vi "Helmholtz2D_FEM_Solve U.vi"(8 "error in (no error)":errorcluster, 11 "Helmholtz2D FEM Data In":T1) -> (0 "error out":errorcluster, 3 "Helmholtz2D FEM Data Out":T1)   [LabVIEW 2017, in "NI_PDE.lvlib"]
uses:
  <vilib>/gmath/NI_PDE.lvlib
  <vilib>/gmath/pde.llb/Helmholtz2D_FEM/Helmholtz2D_FEM_Data.ctl
  <vilib>/gmath/pde.llb/Common/PDE_Sparse Mtrx.ctl
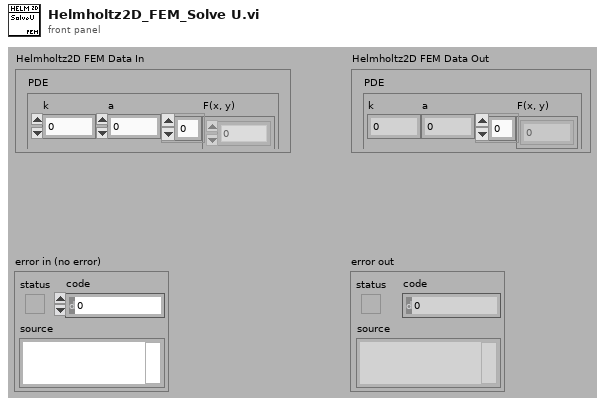
[diagram p1: front panel]
types:
  T1 = typedef "NI_PDE.lvlib/Helmholtz2D_FEM_Data.ctl" = cluster{"PDE":cluster{"k":dbl, "a":dbl, "F(x, y)":dbl[]}, "# of unknown":i32, "# of known":i32, "U(x, y)":dbl[], "X Used":dbl[], "Y Used":dbl[], "Triangulation":i32[][], "Coef Mtrx":T2}
  T2 = typedef "NI_PDE.lvlib/PDE_Sparse Mtrx.ctl" = cluster{"Row":cluster{"col":i32, "value":dbl}[]}[]
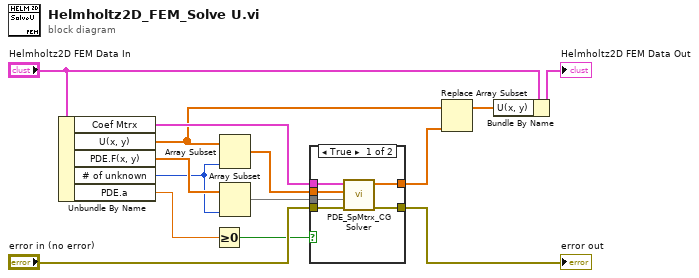
[diagram p0: block diagram]
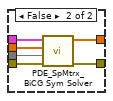
[diagram p2: hidden frame]
diagram:
  n1 = Unbundle By Name("Helmholtz2D FEM Data In") -> ("Coef Mtrx"=w14:T2, "U(x, y)"=w9:dbl[], "PDE.F(x, y)"=w12:dbl[], "# of unknown"=w11:i32, "PDE.a"=w2:dbl)
  n2 = Greater Or Equal To 0?(x=w2) -> (x >= 0?=w1:bool)
  n3 = Array Subset(array=w9, length=w11) -> (w13:dbl[])  [unwired: 1 in]
  n4 = Array Subset(array=w12, length=w11) -> (w10:dbl[])  [unwired: 1 in]
  n5 = case shown="True" w1 {
    tunnel: w14 -> [w20 w26]
    tunnel: w13 -> [w19 w25]
    tunnel: w10 -> [w15 w21]
    tunnel: [w18 w24] -> w8
    tunnel: "error in (no error)" -> [w17 w23]
    tunnel: [w16 w22] -> w3
    frame True {
      n6 = call <vilib>:"PDE_SpMtrx_CG Solver.vi"("error in (no error)"=w17, "X0"=w15, "RHS"=w19, "Sparse Mtrx"=w20) -> ("error out"=w16:errorcluster, "X"=w18:dbl[])  [unwired: 1 in, 5 out]
    }
    frame False {
      n7 = call <vilib>:"PDE_SpMtrx_BiCG Sym Solver.vi"("error in (no error)"=w23, "X0"=w21, "RHS"=w25, "Sparse Mtrx"=w26) -> ("error out"=w22:errorcluster, "X"=w24:dbl[])  [unwired: 1 in, 5 out]
    }
  }
  "error out" <- w3
  n8 = Replace Array Subset(array=w9, new element=w8) -> (w6:dbl[])  [unwired: 1 in]
  n9 = Bundle By Name(cluster="Helmholtz2D FEM Data In", "U(x, y)"=w6) -> (→"Helmholtz2D FEM Data Out":T1)
